vi "EventLogger.vi"(8 "Error In":errorcluster, 11 "EventLoggerQueue":refnum<queue>) -> (0 "Error Out":errorcluster)   [LabVIEW 2019, in "EventLogger.lvlib"]
uses:
  EventLogger.lvlib
  Cluster - MessageCluster.ctl
  Enum - Message.ctl
  Cluster - EventLoggerData.ctl
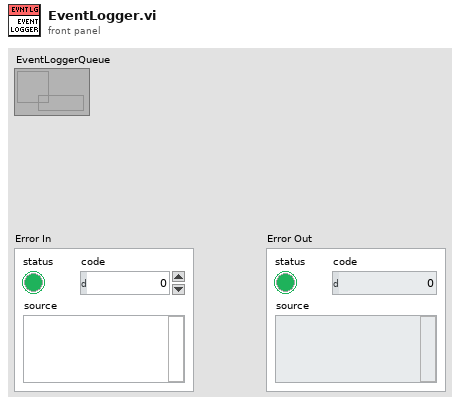
[diagram p1: front panel]
types:
  T1 = typedef "EventLogger.lvlib/Cluster - EventLoggerData.ctl" = cluster{"LogPath":path, "LogRef":refnum<file>}
  T2 = typedef "EventLogger.lvlib/Enum - Message.ctl" = enum16{"Initialize", "Idle", "CreateLog", "LogStrEvent", "LogErrorEvent", "LogVICall", "Error", "Exit"}
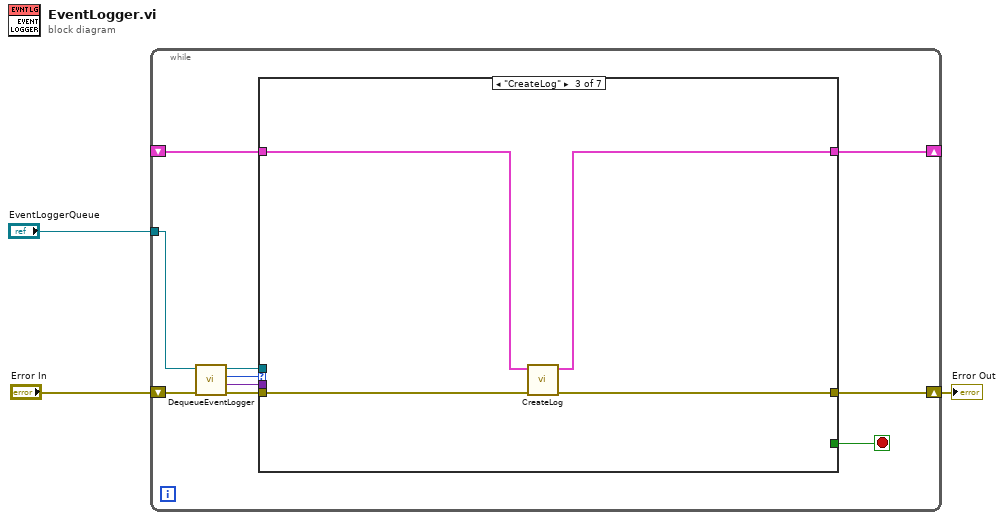
[diagram p0: block diagram]
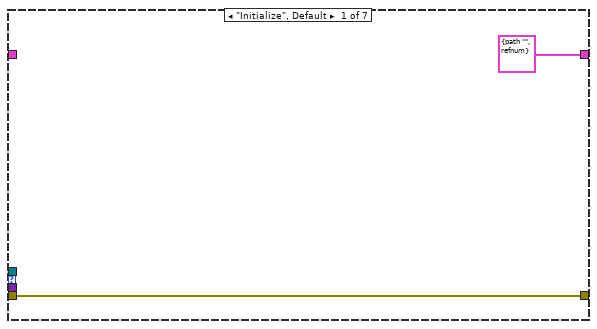
[diagram p2: hidden frame]
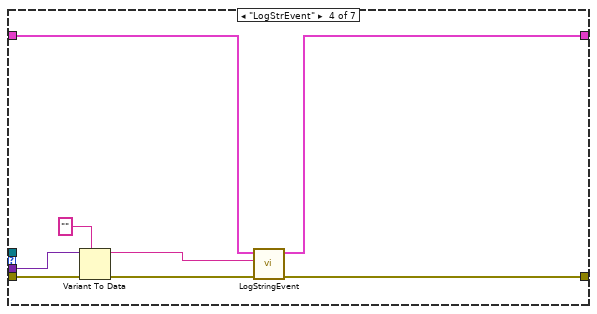
[diagram p4: hidden frame]
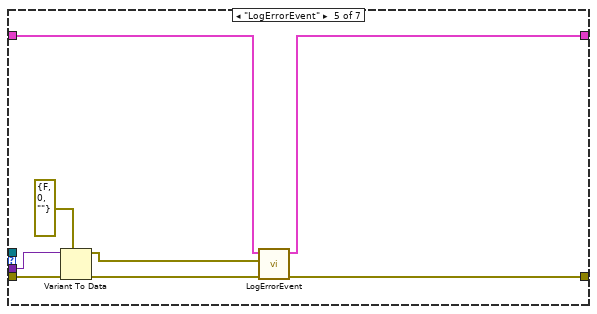
[diagram p5: hidden frame]
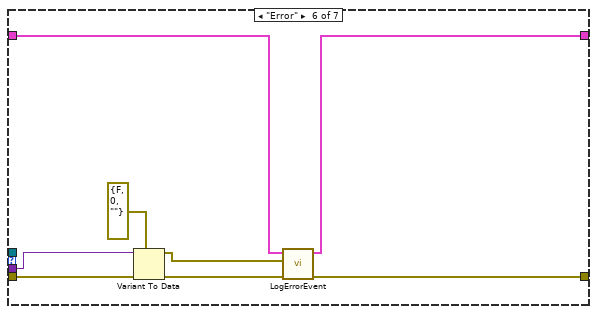
[diagram p6: hidden frame]
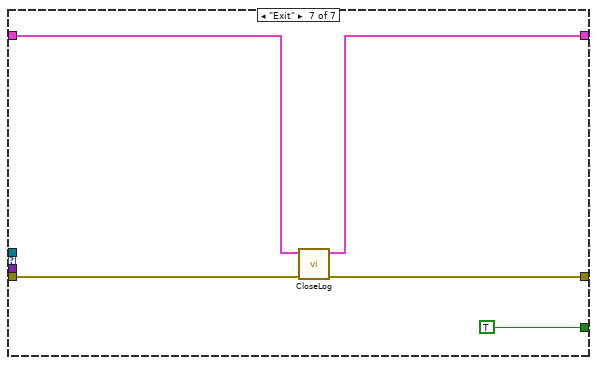
[diagram p7: hidden frame]
diagram:
  n1 = while {
    tunnel: "EventLoggerQueue" -> [w9]
    shift-right: [w13] -> w3
    shift-left: "Error In" -> [w12]
    shift-right: [w5] -> _
    shift-left: _ -> [w4]
    stop <- w6 stop-if-true
    n2 = call "DequeueEventLogger.vi"("error in (no error)"=w12, "Queue in"=w9) -> ("error out"=w11:errorcluster, "Data"=w7:variant, "Message"=w8:T2, "Queue out"=w10:refnum<queue>)  [unwired: 6 in]
    n3 = case shown="\"CreateLog\"" w8 {
      tunnel: [w15 w17 w20 w23 w34 w45 w47] -> w13
      tunnel: w11 -> [w15 w17 w21 w29 w35 w42 w50]
      tunnel: w10 -> [_ _ _ _ _ _ _]
      tunnel: w7 -> [_ _ _ w28 w32 w40 _]
      tunnel: [_ _ _ _ _ _ TRUE] -> w6
      tunnel: [T1 {"LogPath"=path "", "LogRef"=refnum} ("EventLoggerData") w16 w19 w26 w37 w43 w46] -> w5
      tunnel: w4 -> [_ w16 w18 w25 w36 w44 w48]
      frame "Initialize", Default {
      }
      frame "Idle" {
      }
      frame "CreateLog" {
        n4 = call "CreateLog.vi"("error in (no error)"=w21, "EventLoggerData in"=w18) -> ("error out"=w20:errorcluster, "EventLoggerData out"=w19:T1)  [unwired: 8 in]
      }
      frame "LogStrEvent" {
        n5 = Variant To Data(error in=w29, type="", Variant=w28) -> (data=w22:string, error out=w24:errorcluster)
        n6 = call "LogStringEvent.vi"("error in (no error)"=w24, "StringEvent"=w22, "EventLoggerData in"=w25) -> ("error out"=w23:errorcluster, "EventLoggerData out 2"=w26:T1)  [unwired: 7 in]
      }
      frame "LogErrorEvent" {
        n7 = Variant To Data(error in=w35, type=errorcluster {"status"=FALSE, "code"=0, "source"=""} ("error constant"), Variant=w32) -> (data=w30:errorcluster, error out=w33:errorcluster)
        n8 = call "LogErrorEvent.vi"("error in (no error)"=w33, "ErrorEvent"=w30, "EventLoggerData in"=w36) -> ("error out"=w34:errorcluster, "EventLoggerData out 3"=w37:T1)  [unwired: 7 in]
      }
      frame "Error" {
        n9 = Variant To Data(error in=w42, type=errorcluster {"status"=FALSE, "code"=0, "source"=""} ("error out"), Variant=w40) -> (data=w38:errorcluster, error out=w41:errorcluster)
        n10 = call "LogErrorEvent.vi"("error in (no error)"=w41, "ErrorEvent"=w38, "EventLoggerData in"=w44) -> ("error out"=w45:errorcluster, "EventLoggerData out 3"=w43:T1)  [unwired: 7 in]
      }
      frame "Exit" {
        n11 = call "CloseLog.vi"("error in (no error)"=w50, "EventLoggerData out 4"=w48) -> ("error out"=w47:errorcluster, "EventLoggerData out 3"=w46:T1)  [unwired: 8 in]
      }
    }
  }
  "Error Out" <- w3
